vi "Finish.vi"(8 "error in (no error)":errorcluster, 11 "Comp Pressure in":refnum<class "Comp Pressure.lvclass">) -> (0 "error out":errorcluster, 3 "Comp Pressure out":refnum<class "Comp Pressure.lvclass">)   [LabVIEW 2014, in "Comp Pressure.lvlib" / "Comp Pressure.lvclass"]
uses:
  Comp Pressure.lvclass
  Comp Pressure.lvclass/Comp Pressure.ctl
  Robot/Pressure/Pressure Class/Pressure.lvclass
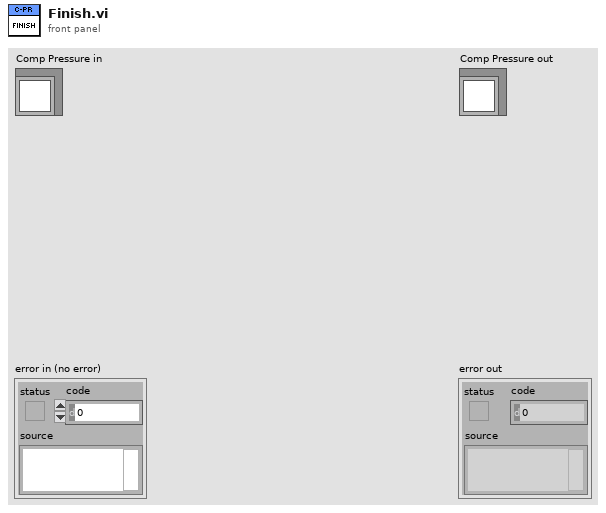
[diagram p1: front panel]
types:
  T1 = typedef "WPI_CompressorDevRef.ctl" = cluster{"DevStatus":errorcluster, "Pneumatics Control Module":u8}
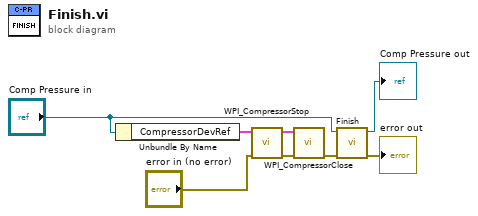
[diagram p0: block diagram]
diagram:
  n1 = Unbundle By Name("Comp Pressure in") -> ("CompressorDevRef"=w5:T1)
  n2 = call <vilib>:"WPI_CompressorStop.vi"("error in (no error)"="error in (no error)", "CompressorDevRef"=w5) -> ("error out"=w2:errorcluster, "CompressorDevRef"=w4:T1)  [unwired: 8 in]
  n3 = call <vilib>:"WPI_CompressorClose.vi"("error in (no error)"=w2, "CompressorDevRef"=w4) -> ("error out"=w1:errorcluster)  [unwired: 9 in]
  n4 = call-parent "Finish.vi"("error in (no error)"=w1, "System Actor in"="Comp Pressure in") -> ("error out"=→"error out":errorcluster, "System Actor out"=→"Comp Pressure out":refnum<class "Comp Pressure.lvclass">)  [unwired: 8 in]
